vi "build_packet.vi"(10 "Packet number":i8, 11 "message data":i8[](array[numeric])) -> (3 "output bitstream":i8[](array[numeric]))   [LabVIEW 2014]
uses:
  <vilib>/addons/Modulation/Digital/General/MT Generate Bits (Galois, PN Order).vi
  <vilib>/addons/Modulation/Digital/Support/Common/Validators/mod_Generate Bits Validate.vi
  <vilib>/addons/Modulation/Analog/support/mod_Set Error Source.vi
  <vilib>/addons/Modulation/Digital/General/subVIs/mod_Generate Bits PN Sequence.vi
  <vilib>/addons/Modulation/niDMT.lvlib
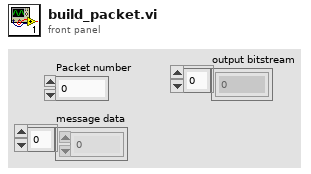
[diagram p1: front panel]
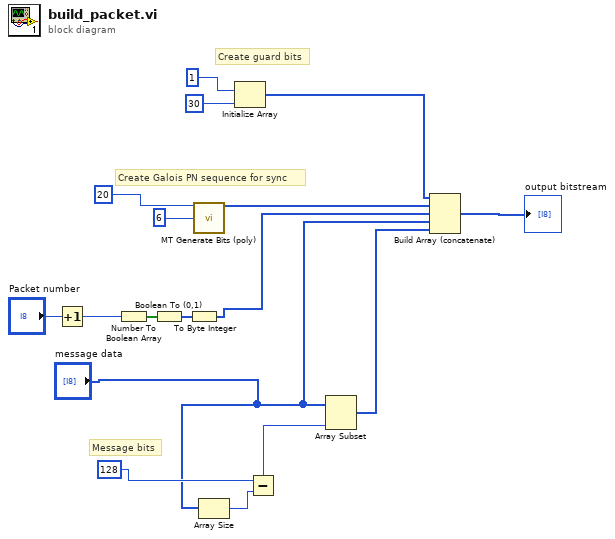
[diagram p0: block diagram]
diagram:
  # "Message bits"
  # "Create Galois PN sequence for sync"
  # "Create guard bits"
  n1 = Increment(x="Packet number") -> (x+1=w3:i8)
  n2 = Number To Boolean Array(number=w3) -> (Boolean array=w4:bool[])
  n3 = Boolean To (0,1)(Boolean=w4) -> (0, 1=w5:i16[])
  n4 = To Byte Integer(number=w5) -> (8bit integer=w2:i8[])
  n5 = call-poly <vilib>:"MT Generate Bits (poly).vi"("total bits (128)"=20, "PN sequence order (9)"=6) -> ("output bit stream"=w12:i8[])  [unwired: 3 in, 10 out]
  n6 = Array Size(array="message data") -> (size(s)=w10:i32)
  n7 = Initialize Array(i8 1 ("element"), 30 ("dimension size")) -> (w13:i8[])
  n8 = Subtract(x=128, y=w10) -> (x-y=w8:i32)
  n9 = Array Subset(array="message data", length=w8) -> (w11:i8[])  [unwired: 1 in]
  n10 = Build Array (concatenate)(w13, w12, w2, "message data", w11) -> (→"output bitstream":i8[])
